vi "Reset ChanCfg.vi"(8 "error in (no error)":errorcluster, 10 "Timing Engine":T1, 11 "Channel in":refnum<class "Channel.lvclass">) -> (0 "error out":errorcluster, 3 "Channel out":refnum<class "Channel.lvclass">)   [LabVIEW 2018, in "Measurement Channels.lvlib" / "Channel.lvclass"]
uses:
  Channel.lvclass
  Common/Controls/TE_Designator.ctl
  Channel.lvclass/Channel.ctl
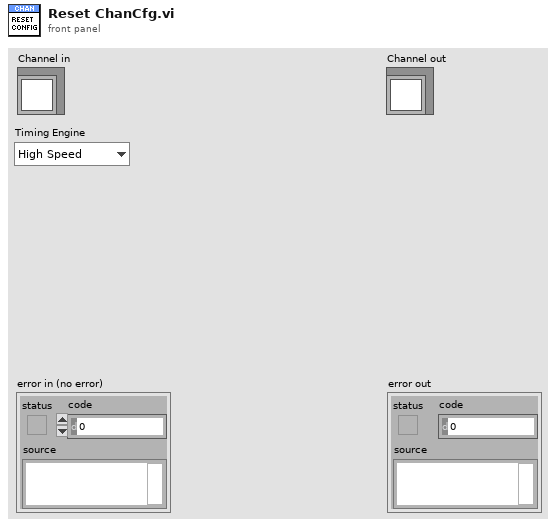
[diagram p1: front panel]
types:
  T1 = typedef "TE_Designator.ctl" = enum16{"High Speed", "Low Speed"}
  T2 = typedef "DAQMan Definitions.ctl" = cluster{"Timing Engine Defs":variant, "Table Definitions":variant, "Ring Definitions":variant}
  T3 = typedef "HeaderNames.ctl" = enum16{"Channel", "Device", "Spacer", "Description", "MB", "Range", "Terminal", "Coupling", "Thresh (V)", "Pulse/Rev", "Slope", "Min EU", "Min RPM", "mV/EU", "Iex", "Temp Units", "Type", "CJC Src", "CJC Val", "Ro", "Wire Cfg", "Strain Mode", "Vex", "Bridge Type", "GF", "Gauge Res", "Poisson", "Lead Res", "Init Strain", "GAF", "Scale", "Offset", "Unit (EU)", "dB?", "dB Ref", "Cal Mag", "Cal Units", "Max Temp", "Min Temp", "Max Strain", "Min Strain"}
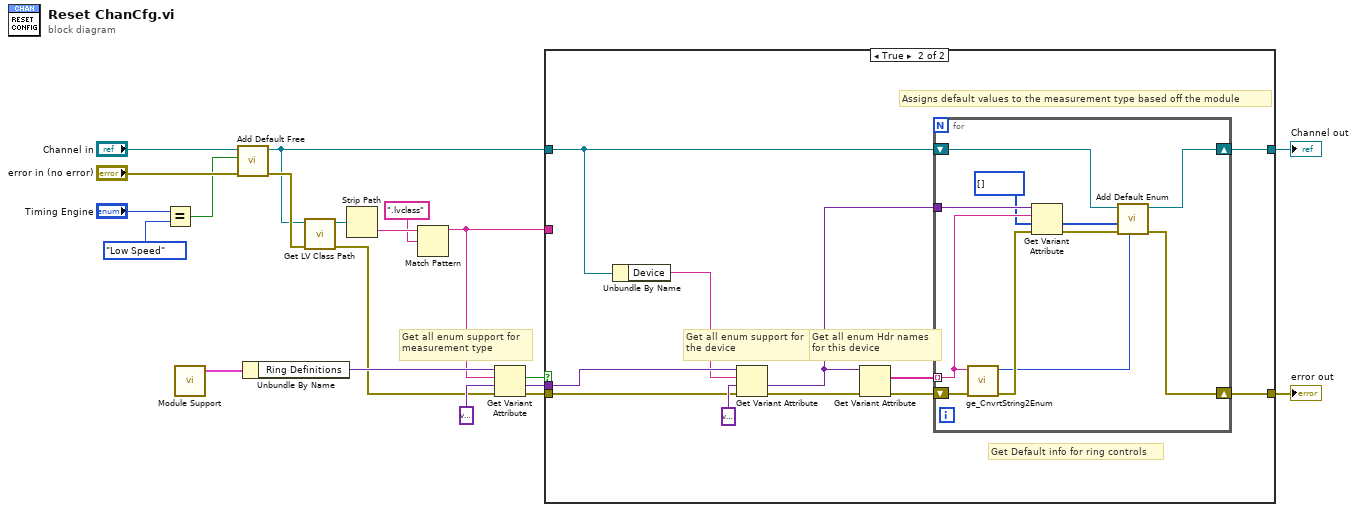
[diagram p0: block diagram]
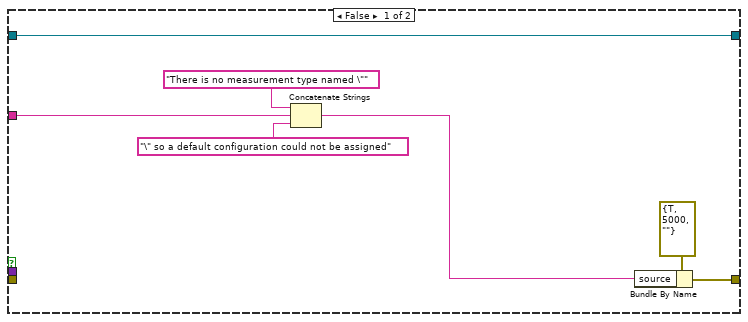
[diagram p2: hidden frame]
diagram:
  # "Get all enum support for\nmeasurement type"
  n1 = Equal?(x="Timing Engine", y=TE_Designator."Low Speed") -> (x = y?=w2:bool)
  n2 = call "Module Support.vi"() -> ("ge_DAQManDefinitions"=w1:T2)  [unwired: 9 in]
  n3 = call-dynamic "Add Default Free.vi"("error in (no error)"="error in (no error)", "ToModBus"=w2, "Channel in"="Channel in") -> ("error out"=w10:errorcluster, "Channel out"=w9:refnum<class "Channel.lvclass">)  [unwired: 7 in]
  n4 = Unbundle By Name(w1) -> ("Ring Definitions"=w18:variant)
  n5 = call <vilib>:"Get LV Class Path.vi"("error in (no error)"=w10, "object"=w9) -> ("error out"=w11:errorcluster, "class path"=w12:path)  [unwired: 8 in]
  n6 = Strip Path(path=w12) -> (name=w8:string)  [unwired: 1 out]
  n7 = Match Pattern(string=w8, regular expression=".lvclass") -> (before substring=w5:string)  [unwired: 1 in, 3 out]
  n8 = Get Variant Attribute(Variant=w18, name=w5, default value (empty Variant)=variant ("All Ring Support"), error in=w11) -> (found=w6:bool, value=w16:variant, error out=w17:errorcluster)  [unwired: 1 out]
  n9 = case shown="True" w6 {
    tunnel: [w27 w38] -> w19
    tunnel: w17 -> [_ w30]
    tunnel: w16 -> [_ w36]
    tunnel: [w25 w31] -> w14
    tunnel: w9 -> [w27 w29]
    tunnel: w5 -> [w24 _]
    frame False {
      n10 = Concatenate Strings("There is no measurement type named \"" ("string"), w24, "\" so a default configuration could not be assigned" ("string")) -> (w21:string)
      n11 = Bundle By Name(cluster=errorcluster {"status"=TRUE, "code"=5000, "source"=""} ("error out"), "source"=w21) -> (w25:errorcluster)
    }
    frame True {
      # "Get all enum support for\nthe device"
      # "Get all enum Hdr names\nfor this device"
      # "Assigns default values to the measurement type based off the module"
      # "Get Default info for ring controls"
      n12 = Unbundle By Name(w29) -> ("Device"=w28:string)
      n13 = Get Variant Attribute(Variant=w36, name=w28, default value (empty Variant)=variant ("All Ring Support"), error in=w30) -> (value=w37:variant, error out=w33:errorcluster)  [unwired: 2 out]
      n14 = Get Variant Attribute(Variant=w37, error in=w33) -> (names=w35:string[], error out=w34:errorcluster)  [unwired: 2 in, 2 out]
      n15 = for {
        tunnel: w37 -> [w48]
        shift-right: [w41] -> w31
        shift-left: w34 -> [w49]
        tunnel: w35 -> [w46] mode=indexing
        shift-right: [w43] -> w38
        shift-left: w29 -> [w44]
        n16 = call "ge_CnvrtString2Enum.vi"("error in (no error)"=w49, "Enum String"=w46) -> ("error out"=w47:errorcluster, "Hdr Name"=w40:T3)  [unwired: 8 in]
        n17 = Get Variant Attribute(Variant=w48, name=w46, default value (empty Variant)=u16[] [] ("Values"), error in=w47) -> (value=w39:u16[], error out=w42:errorcluster)  [unwired: 2 out]
        n18 = call-dynamic "Add Default Enum.vi"("Hdr Name"=w40, "error in (no error)"=w42, "Enum Values"=w39, "Channel in"=w44) -> ("error out"=w41:errorcluster, "Channel out"=w43:refnum<class "Channel.lvclass">)  [unwired: 6 in]
      }
    }
  }
  "Channel out" <- w19
  "error out" <- w14
